vi "Calculate delta hue with wrap around.vi"(9 "Hue.Mean 2":u8=200, 11 "Hue.Mean 1":u8=5) -> (2 "Hue delta":u8=61)   [LabVIEW 2013]
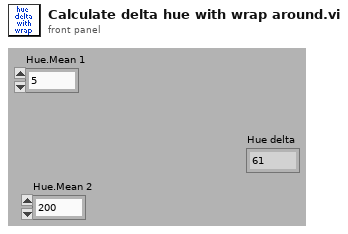
[diagram p1: front panel]
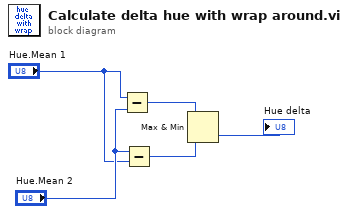
[diagram p0: block diagram]
diagram:
  n1 = Subtract(x="Hue.Mean 1", y="Hue.Mean 2") -> (x-y=w3:u8)
  n2 = Subtract(x="Hue.Mean 2", y="Hue.Mean 1") -> (x-y=w2:u8)
  n3 = Max & Min(x=w3, y=w2) -> (min(x,y)=→"Hue delta":u8)  [unwired: 1 out]
